vi "Cam_Init_Done.vi"(8 "error in (no error)":errorcluster, 10 "Variant":variant, 11 "Cam_SLM_Controller in":refnum<class "Cam_SLM_Controller.lvclass">) -> (0 "error out":errorcluster, 3 "Cam_SLM_Controller out":refnum<class "Cam_SLM_Controller.lvclass">)   [LabVIEW 2023, in "Cam_SLM_controller.lvlib" / "Cam_SLM_Controller.lvclass"]
uses:
  Cam_SLM_Controller.lvclass
  Cam_SLM_Controller.lvclass/Cam_SLM_Controller.ctl
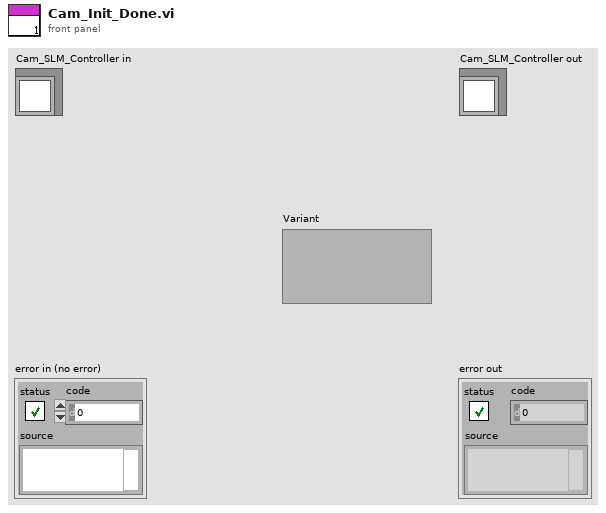
[diagram p1: front panel]
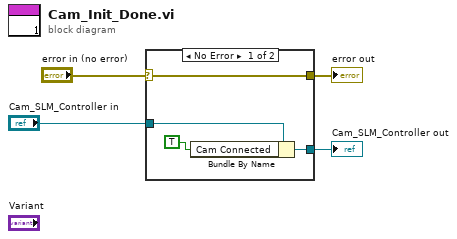
[diagram p0: block diagram]
diagram:
  n1 = case shown="No Error" "error in (no error)" {
    selector: "error in (no error)" -> [w8 w10]
    tunnel: [w8 w10] -> w1
    tunnel: [w5 w9] -> w3
    tunnel: "Cam_SLM_Controller in" -> [w7 w9]
    frame No Error {
      n2 = Bundle By Name(cluster=w7, "Cam Connected"=TRUE) -> (w5:refnum<class "Cam_SLM_Controller.lvclass">)
    }
    frame Error {
    }
  }
  "error out" <- w1
  "Cam_SLM_Controller out" <- w3
